vi "calc_lookup_arrays.vi"(8 "error in":errorcluster, 9 "Pixels per spiral":T1=1 min=1 max=90000 step=1, 10 "All scan parameters":T2={"Fiber parameters"={"Frequency"=100.0, "Amplitude X"=0.0, "Amplitude Y"=0.0, "Initial Amplitude X"=0.0, "Initial Amplitude Y"=0.0, "Phase"=0.0}, "Spiral parameters"={"Imaging periods"=1.0, "Settling periods"=1.0, "Resting periods"=1.0}, "Run parameters"={"Run mode"=enum."Continuous", "Averages per frame"=1, "No. of frames"=1}, "Acquisition parameters"={"Cycles per pixel"=0, "Image size"=1, "Bidirectional acquisition"=FALSE}, "Fiber parameters pixel_mapper"={"Frequency"=1.0, "Amplitude X"=1.0, "Amplitude Y"=1.0, "Initial Amplitude X"=0.0, "Initial Amplitude Y"=0.0, "Phase"=0.0}, "Smooth_coeffs_cluster"={"Coeff 1"=0.0, "Coeff 2"=0.0}, "Storage parameters"={"Autosave"=FALSE, "Path"=path ""}, "Mapping corrections"={"Phase increase"=0.0, "Amplitude correction"=0.0}} {"Smooth_coeffs_cluster"."Coeff 1" min=0.0 max=1.0 step=0.05; "Smooth_coeffs_cluster"."Coeff 2" min=0.0 max=1.0 step=0.05; "Fiber parameters pixel_mapper"."Phase" min=-90.0 max=90.0 step=5.0; "Fiber parameters pixel_mapper"."Initial Amplitude Y" min=0.0 max=1.0 step=0.1; "Fiber parameters pixel_mapper"."Initial Amplitude X" min=0.0 max=1.0 step=0.1; "Fiber parameters pixel_mapper"."Amplitude Y" min=0.0 max=3.0 step=0.1; "Fiber parameters pixel_mapper"."Amplitude X" min=0.0 max=3.0 step=0.1; "Fiber parameters pixel_mapper"."Frequency" min=100.0 max=6000.0 step=1.0; "Acquisition parameters"."Image size" items=["128x128 px"=128, "256x256 px"=256, "512x512 px"=512]; "Acquisition parameters"."Cycles per pixel" min=100 max=90000 step=1; "Run parameters"."No. of frames" min=1 max=1000 step=1; "Run parameters"."Averages per frame" min=1 max=32; "Spiral parameters"."Resting periods" min=10.0 max=1000.0 step=1.0; "Spiral parameters"."Settling periods" min=1.0 max=1000.0 step=1.0; "Spiral parameters"."Imaging periods" min=1.0 max=1000.0 step=1.0; "Fiber parameters"."Phase" min=-90.0 max=90.0 step=5.0; "Fiber parameters"."Initial Amplitude Y" min=0.0 max=1.0 step=0.1; "Fiber parameters"."Initial Amplitude X" min=0.0 max=1.0 step=0.1; "Fiber parameters"."Amplitude Y" min=0.0 max=3.0 step=0.1; "Fiber parameters"."Amplitude X" min=0.0 max=3.0 step=0.1; "Fiber parameters"."Frequency" min=100.0 max=6000.0 step=1.0}, 11 "Lookup arrays in":T12) -> (0 "error out":errorcluster, 1 "Phase corrections":dbl[][](array[numeric]), 2 "Amplitude corrections":dbl[][](array[numeric]), 3 "Lookup arrays out":T12)   [LabVIEW 2011, in "Fiberscope_library.lvlib"]
uses:
  Fiberscope_library.lvlib
  typedefs/lookup_arrays_ref_cluster.ctl
  typedefs/all_scan_parameters_cluster.ctl
  typedefs/fiber_parameters_cluster.ctl
  typedefs/spiral_parameters_cluster.ctl
  typedefs/run_parameters_cluster.ctl
  typedefs/run_mode_enum.ctl
  typedefs/acquisition_parameters_cluster.ctl
  typedefs/image_size_I32.ctl
  typedefs/smooth_coeffs_cluster.ctl
  typedefs/storage_parameters_cluster.ctl
  typedefs/mapping_corrections_cluster.ctl
  typedefs/pixel_per_spiral_I32.ctl
  typedefs/lookup_array_parameter_cluster.ctl
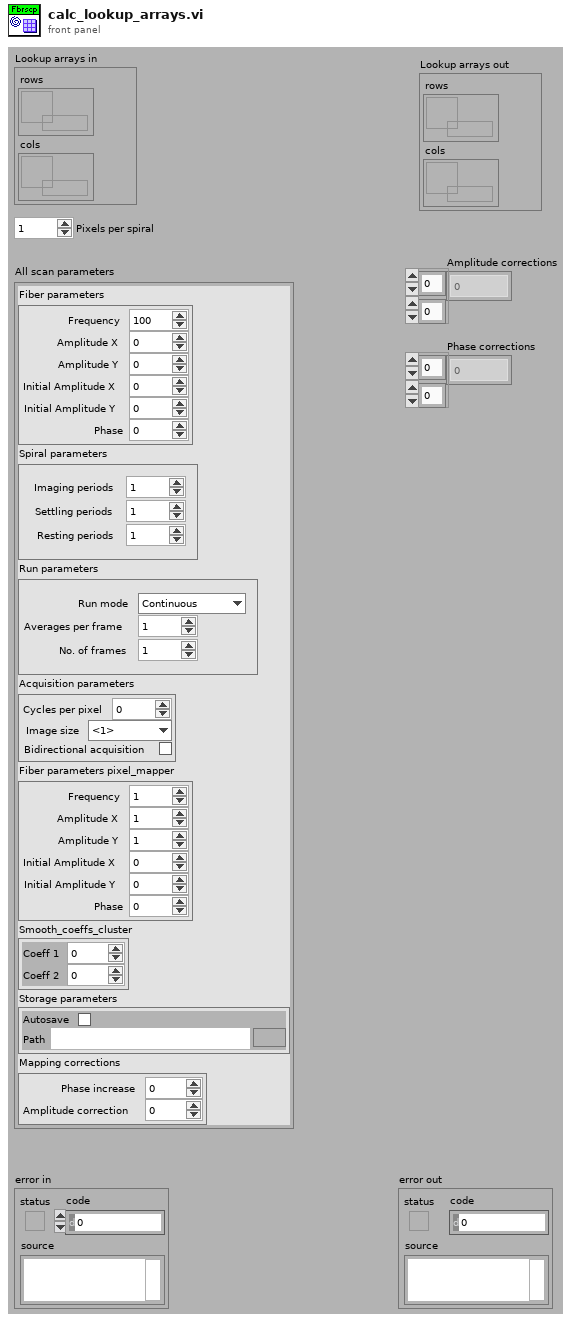
[diagram p1: front panel]
types:
  T1 = typedef "Fiberscope_library.lvlib/pixel_per_spiral_I32.ctl" = i32
  T2 = typedef "Fiberscope_library.lvlib/all_scan_parameters_cluster.ctl" = cluster{"Fiber parameters":T3, "Spiral parameters":T4, "Run parameters":T5, "Acquisition parameters":T7, "Fiber parameters pixel_mapper":T3, "Smooth_coeffs_cluster":T9, "Storage parameters":T10, "Mapping corrections":T11}
  T3 = typedef "Fiberscope_library.lvlib/fiber_parameters_cluster.ctl" = cluster{"Frequency":dbl, "Amplitude X":dbl, "Amplitude Y":dbl, "Initial Amplitude X":dbl, "Initial Amplitude Y":dbl, "Phase":dbl}
  T4 = typedef "Fiberscope_library.lvlib/spiral_parameters_cluster.ctl" = cluster{"Imaging periods":dbl, "Settling periods":dbl, "Resting periods":dbl}
  T5 = typedef "Fiberscope_library.lvlib/run_parameters_cluster.ctl" = cluster{"Run mode":T6, "Averages per frame":u8, "No. of frames":u32}
  T6 = typedef "Fiberscope_library.lvlib/run_mode_enum.ctl" = enum16{"Continuous", "Single frame", "No. of frames"}
  T7 = typedef "Fiberscope_library.lvlib/acquisition_parameters_cluster.ctl" = cluster{"Cycles per pixel":u32, "Image size":T8, "Bidirectional acquisition":bool}
  T8 = typedef "Fiberscope_library.lvlib/image_size_I32.ctl" = i32
  T9 = typedef "Fiberscope_library.lvlib/smooth_coeffs_cluster.ctl" = cluster{"Coeff 1":dbl, "Coeff 2":dbl}
  T10 = typedef "Fiberscope_library.lvlib/storage_parameters_cluster.ctl" = cluster{"Autosave":bool, "Path":path}
  T11 = typedef "Fiberscope_library.lvlib/mapping_corrections_cluster.ctl" = cluster{"Phase increase":dbl, "Amplitude correction":dbl}
  T12 = typedef "Fiberscope_library.lvlib/lookup_arrays_ref_cluster.ctl" = cluster{"rows":refnum<data-value>, "cols":refnum<data-value>}
  T13 = typedef "Fiberscope_library.lvlib/lookup_array_parameter_cluster.ctl" = cluster{"Image size offset":dbl, "Image size scaler":dbl, "Amplitude increment per pixel":dbl, "Initial Amplitude":dbl, "Pixels per spiral":T1, "Period fraction per pixel":dbl, "Initial phase":dbl}
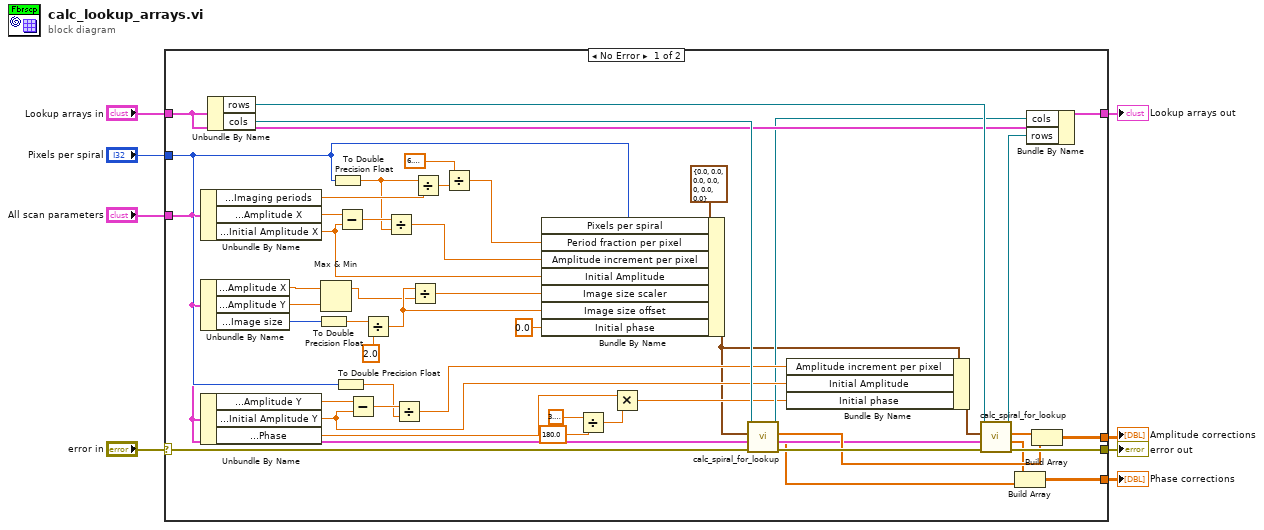
[diagram p0: block diagram]
diagram:
  n1 = case shown="No Error" "error in" {
    selector: "error in" -> [w45 w58]
    tunnel: [w37 w58] -> w7
    tunnel: "All scan parameters" -> [w12 _]
    tunnel: "Lookup arrays in" -> [w29 w57]
    tunnel: [w26 w57] -> w5
    tunnel: "Pixels per spiral" -> [w17 _]
    tunnel: [w13 _] -> w2
    tunnel: [w9 _] -> w1
    frame No Error {
      n2 = Unbundle By Name(w12) -> ("Spiral parameters.Imaging periods"=w55:dbl, "Fiber parameters pixel_mapper.Amplitude X"=w53:dbl, "Fiber parameters pixel_mapper.Initial Amplitude X"=w41:dbl)
      n3 = Unbundle By Name(w12) -> ("Fiber parameters pixel_mapper.Amplitude X"=w50:dbl, "Fiber parameters pixel_mapper.Amplitude Y"=w49:dbl, "Acquisition parameters.Image size"=w48:T8)
      n4 = Unbundle By Name(w12) -> ("Fiber parameters pixel_mapper.Amplitude Y"=w36:dbl, "Fiber parameters pixel_mapper.Initial Amplitude Y"=w32:dbl, "Fiber parameters pixel_mapper.Phase"=w21:dbl)
      n5 = Unbundle By Name(w29) -> ("rows"=w30:refnum<data-value>, "cols"=w39:refnum<data-value>)
      n6 = To Double Precision Float(number=w48) -> (double precision float=w47:dbl)
      n7 = Max & Min(x=w50, y=w49) -> (max(x,y)=w18:dbl)  [unwired: 1 out]
      n8 = To Double Precision Float(number=w17) -> (double precision float=w51:dbl)
      n9 = To Double Precision Float(number=w17) -> (double precision float=w34:dbl)
      n10 = Subtract(x=w53, y=w41) -> (x-y=w52:dbl)
      n11 = Subtract(x=w36, y=w32) -> (x-y=w35:dbl)
      n12 = Divide(x=w47, y=2.0) -> (x/y=w19:dbl)
      n13 = Divide(x=w52, y=w51) -> (x/y=w42:dbl)
      n14 = Divide(x=w35, y=w34) -> (x/y=w33:dbl)
      n15 = Divide(x=w19, y=w18) -> (x/y=w40:dbl)
      n16 = Divide(x=w51, y=w55) -> (x/y=w54:dbl)
      n17 = Divide(x=6.283185307179586, y=w54) -> (x/y=w43:dbl)
      n18 = Bundle By Name(cluster=T13 {"Image size offset"=0.0, "Image size scaler"=0.0, "Amplitude increment per pixel"=0.0, "Initial Amplitude"=0.0, "Pixels per spiral"=0, "Period fraction per pixel"=0.0, "Initial phase"=0.0} ("Lookup array parameter cluster"), "Pixels per spiral"=w17, "Period fraction per pixel"=w43, "Amplitude increment per pixel"=w42, "Initial Amplitude"=w41, "Image size scaler"=w40, "Image size offset"=w19, "Initial phase"=0.0) -> (w16:T13)
      n19 = Divide(x=3.141592653589793, y=180.0) -> (x/y=w22:dbl)
      n20 = Multiply(x=w21, y=w22) -> (x*y=w20:dbl)
      n21 = call "calc_spiral_for_lookup.vi"("error in"=w45, "All scan parameters"=w12, "Lookup array parameter cluster"=w16, "Lookup array memref in"=w39) -> ("error out"=w38:errorcluster, "Phase correction"=w10:dbl[], "Amplitude correction"=w14:dbl[], "Lookup array memref out"=w28:refnum<data-value>)  [unwired: 2 in]
      n22 = Bundle By Name(cluster=w16, "Amplitude increment per pixel"=w33, "Initial Amplitude"=w32, "Initial phase"=w20) -> (w31:T13)
      n23 = call "calc_spiral_for_lookup.vi"("error in"=w38, "All scan parameters"=w12, "Lookup array parameter cluster"=w31, "Lookup array memref in"=w30) -> ("error out"=w37:errorcluster, "Phase correction"=w11:dbl[], "Amplitude correction"=w15:dbl[], "Lookup array memref out"=w27:refnum<data-value>)  [unwired: 2 in]
      n24 = Build Array(w11, w10) -> (w9:dbl[][])
      n25 = Bundle By Name(cluster=w29, "cols"=w28, "rows"=w27) -> (w26:T12)
      n26 = Build Array(w15, w14) -> (w13:dbl[][])
    }
    frame Error {
    }
  }
  "error out" <- w7
  "Lookup arrays out" <- w5
  "Amplitude corrections" <- w2
  "Phase corrections" <- w1
